vi "LEO_CONTROL.vi"() -> ()   [LabVIEW 2017]
panel:
  in  "SAVE CURRENT IMAGE":bool
  out "Last Action @":string="12:38:13 PM"
  out "Completion Response  2":string=">SmartSEM Remote Control V04.08, 24th July 2009"
  out "Acknowledge Response 2":string="@"
  in  "ANGLE":dbl=45.0 min=0.0 max=360.0
  in  "ON/OFF":bool
  in  "LINE (Y)":i32=384 min=0 max=767
  in  "Y":i32=384 min=0 max=767
  in  "X":i32=512 min=0 max=1023
  in  "MAG":i32=2000 min=5 max=500000
  in  "RATE":i32(ring)=7 items=["1"=1, "2"=2, "3"=3, "4"=4, "5"=5, "6"=6, "7"=7, "8"=8, "9"=9, "10"=10, "11"=11, "12"=12, "13"=13, "14"=14, "15"=15]
  in  "SCAN ROTATION":bool
  in  "CENTER BEAM":bool
  in  "SET NORMAL MODE":bool
  in  "SET LINE MODE":bool
  in  "SET SPOT MODE":bool
  in  "SET MAG":bool
  in  "SET SCAN RATE":bool
  in  "BLANK BEAM":bool
  in  "ABORT":bool
  out "error out 2":errorcluster
  out "Completion Response":string
  out "Acknowledge Response":string
  in  "VER?":bool
  in  "stop":bool
  out "error out":errorcluster={"status"=FALSE, "code"=0, "source"="Response\nindicates valid\n command."}
  in  "VISA resource name":refnum<visa-resource-name>="COM4"
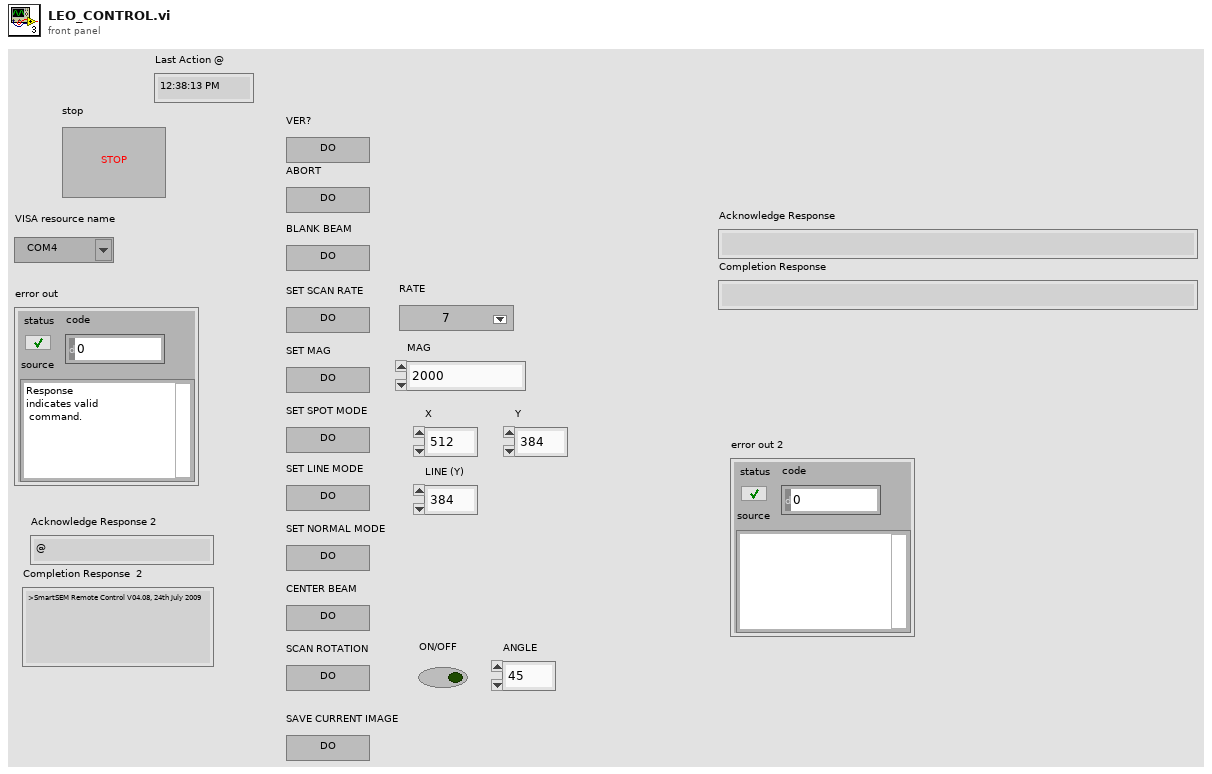
[diagram p1: front panel]
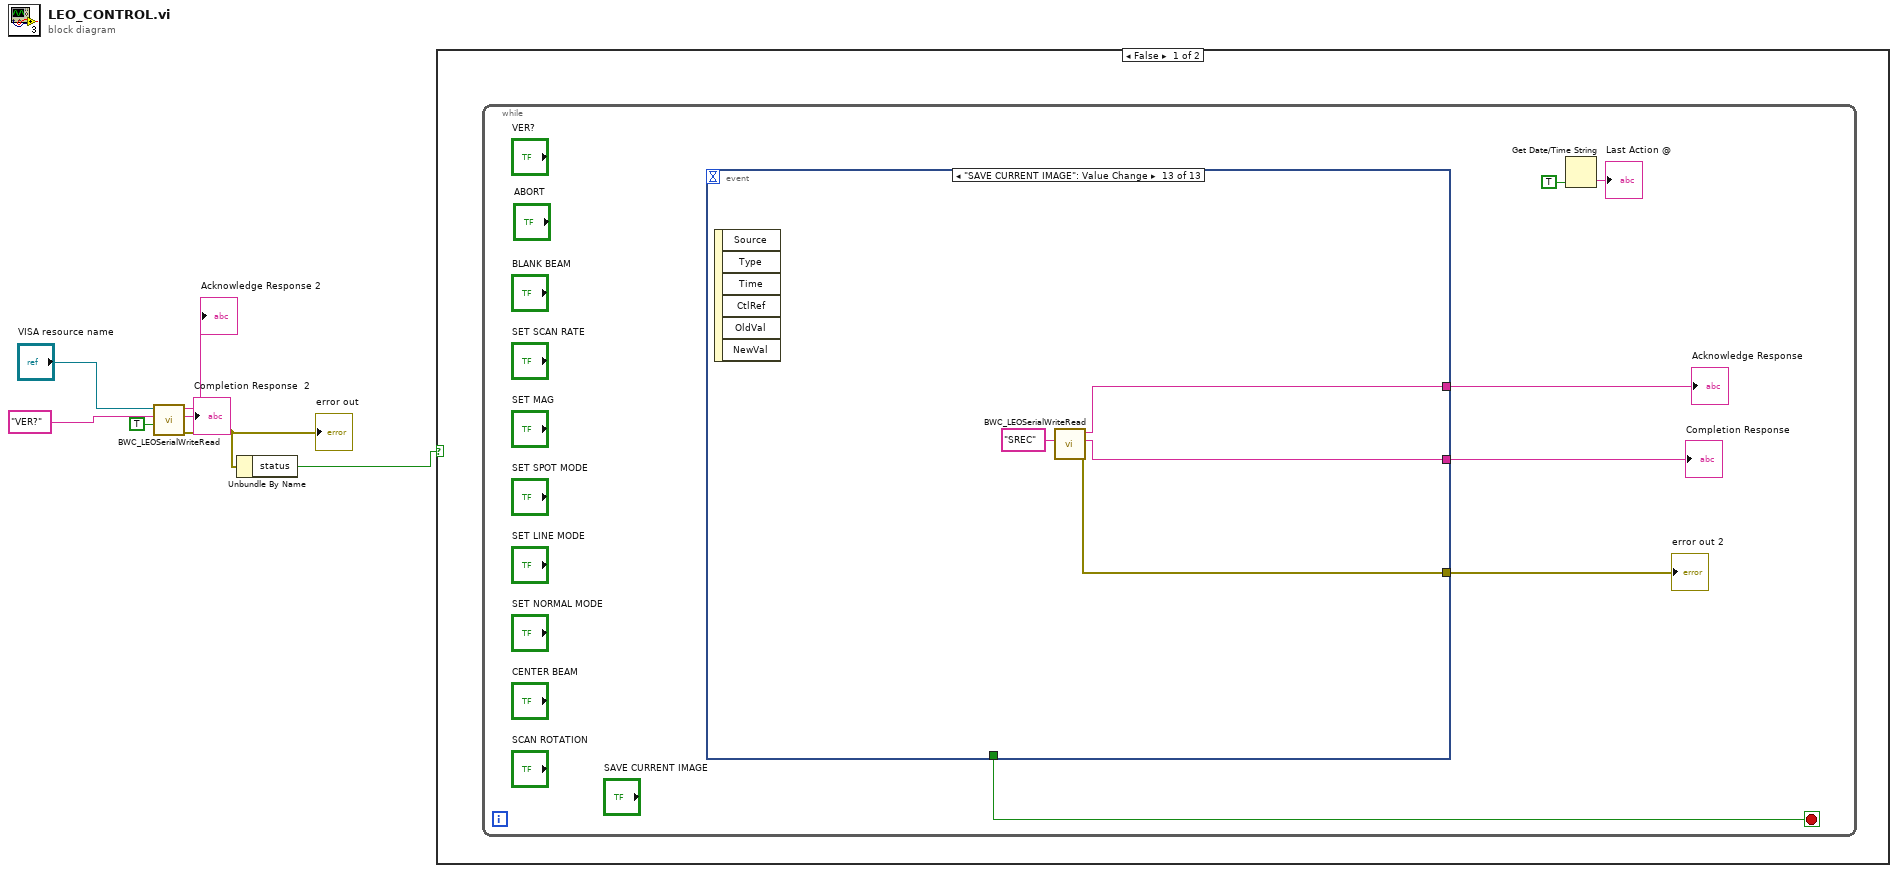
[diagram p0: block diagram]
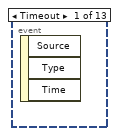
[diagram p2: hidden frame]
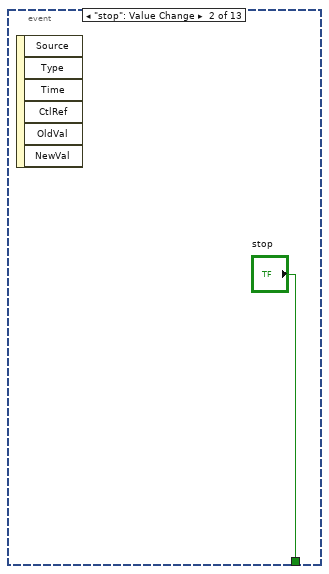
[diagram p3: hidden frame]
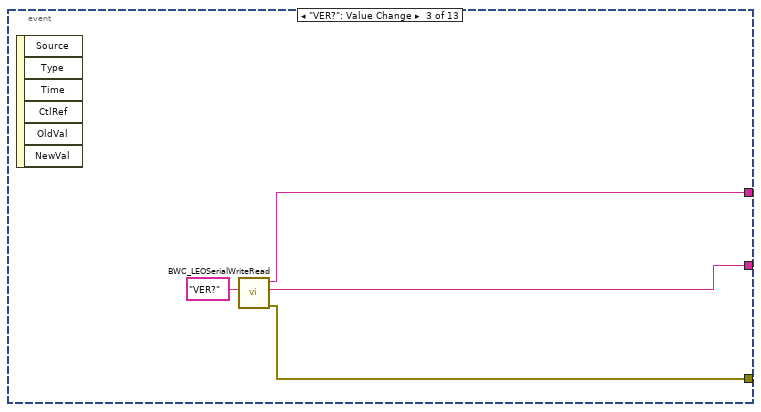
[diagram p4: hidden frame]
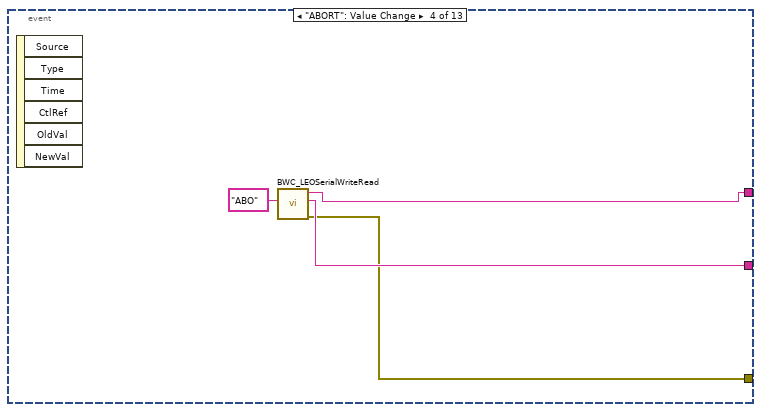
[diagram p5: hidden frame]
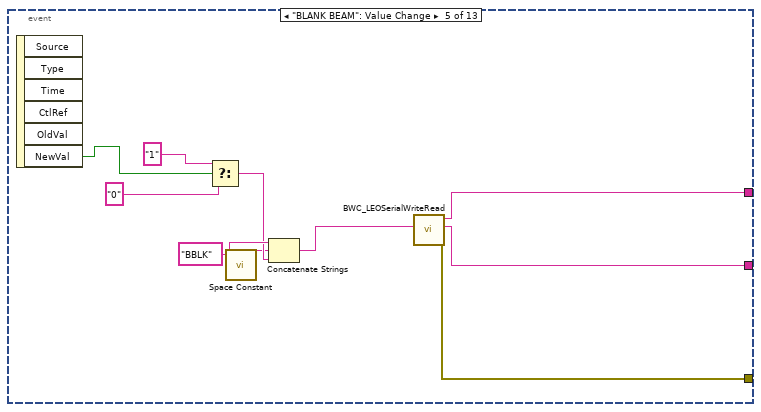
[diagram p6: hidden frame]
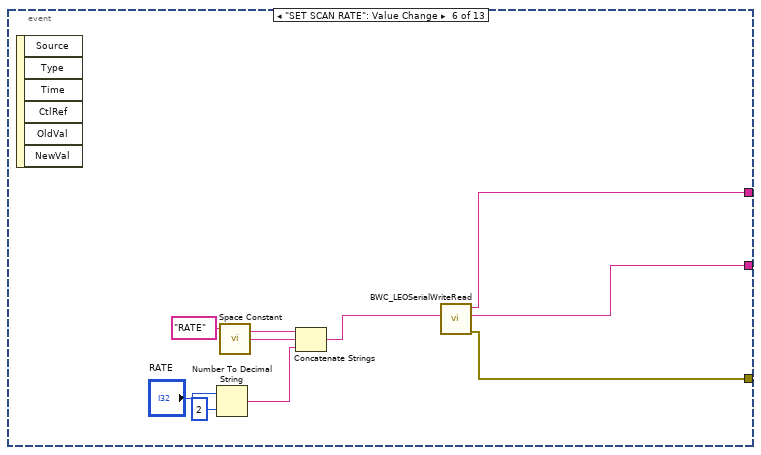
[diagram p7: hidden frame]
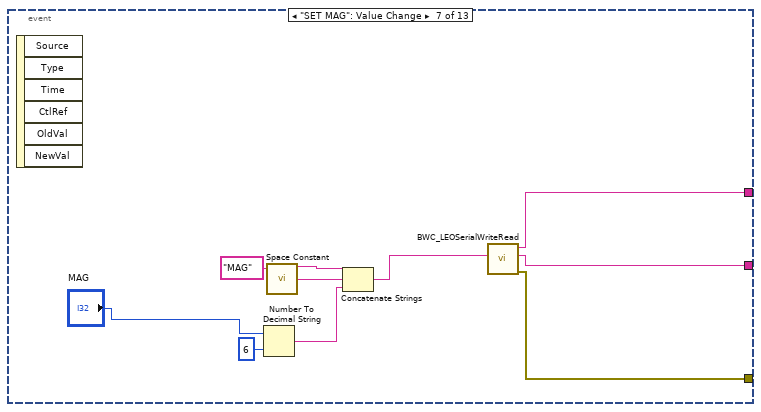
[diagram p8: hidden frame]
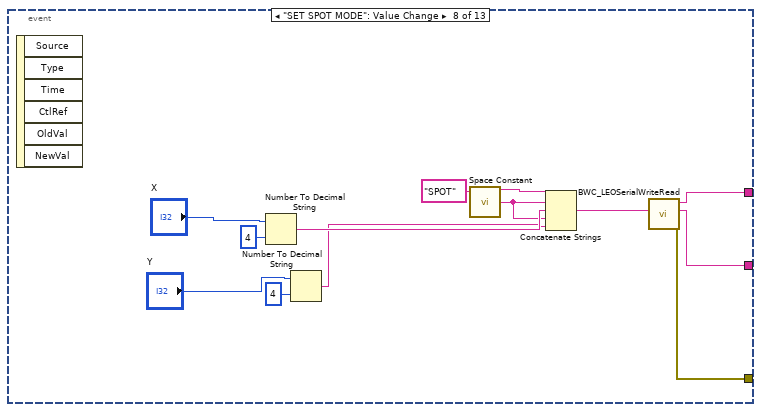
[diagram p9: hidden frame]
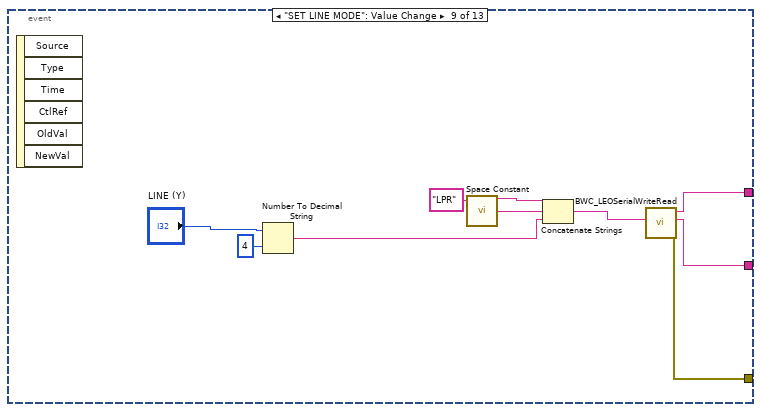
[diagram p10: hidden frame]
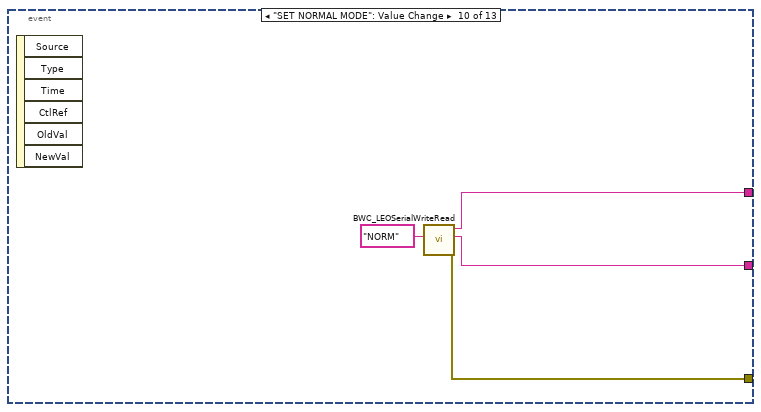
[diagram p11: hidden frame]
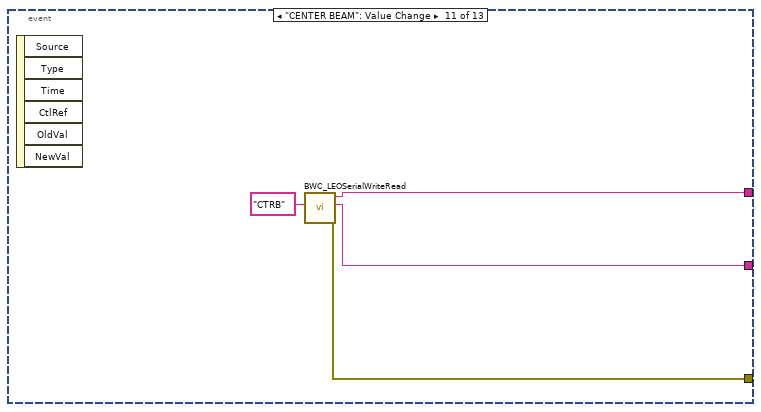
[diagram p12: hidden frame]
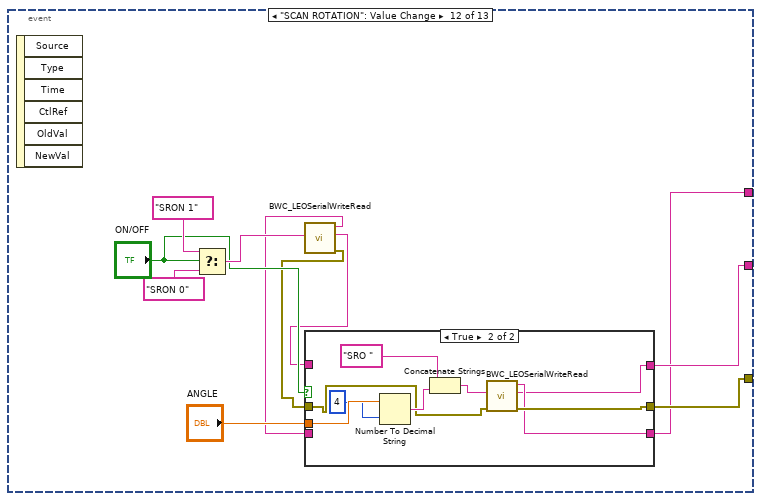
[diagram p13: hidden frame]
diagram:
  n1 = call "BWC_LEOSerialWriteRead.vi"("Perform Two Reads Following Write"=TRUE, "Command To Write"="VER?", "VISA resource name"="VISA resource name") -> ("error out"=w4:errorcluster, "Completion Response"=→"Completion Response  2":string, "Acknowledge Response"=→"Acknowledge Response 2":string)  [unwired: 4 in, 1 out]
  "error out" <- w4
  n2 = Unbundle By Name(w4) -> ("status"=w3:bool)
  n3 = case shown="False" w3 {
    frame False {
      n4 = while {
        stop <- w10 stop-if-true
        n5 = event shown="[12] \"SAVE CURRENT IMAGE\": Value Change" {
          selector: _ -> [_ _ _ _ _ _ _ _ _ _ _ _ _]
          dyn-events: _ -> [_ _ _ _ _ _ _ _ _ _ _ _ _]
          timeout: _ -> [_ _ _ _ _ _ _ _ _ _ _ _ _]
          tunnel: [_ _ w17 w21 w25 w35 w43 w59 w65 w74 w78 w81 w105] -> w13
          tunnel: [_ _ w16 w20 w24 w34 w44 w58 w64 w73 w77 w83 w104] -> w12
          tunnel: [_ _ w15 w19 w23 w33 w42 w57 w63 w72 w76 w84 w103] -> w11
          tunnel: [_ "stop" _ _ _ _ _ _ _ _ _ _ _] -> w10
          event Timeout {
            n6 = event-data() -> ()  [unwired: 1 in, 3 out]
          }
          event "stop": Value Change {
            n7 = event-data() -> ()  [unwired: 1 in, 6 out]
          }
          event "VER?": Value Change {
            n8 = event-data() -> ()  [unwired: 1 in, 6 out]
            n9 = call "BWC_LEOSerialWriteRead.vi"("Command To Write"="VER?") -> ("error out"=w15:errorcluster, "Completion Response"=w16:string, "Acknowledge Response"=w17:string)  [unwired: 6 in, 1 out]
          }
          event "ABORT": Value Change {
            n10 = event-data() -> ()  [unwired: 1 in, 6 out]
            n11 = call "BWC_LEOSerialWriteRead.vi"("Command To Write"="ABO") -> ("error out"=w19:errorcluster, "Completion Response"=w20:string, "Acknowledge Response"=w21:string)  [unwired: 6 in, 1 out]
          }
          event "BLANK BEAM": Value Change {
            n12 = event-data() -> ("NewVal"=w32:bool)  [unwired: 1 in, 5 out]
            n13 = Select(t="1", s=w32, f="0") -> (s? t:f=w28:string)
            n14 = call <vilib>:"Space Constant.vi"() -> ("String"=w27:string)
            n15 = Concatenate Strings("BBLK" ("Command To Write"), w27, w28) -> (w26:string)
            n16 = call "BWC_LEOSerialWriteRead.vi"("Command To Write"=w26) -> ("error out"=w23:errorcluster, "Completion Response"=w24:string, "Acknowledge Response"=w25:string)  [unwired: 6 in, 1 out]
          }
          event "SET SCAN RATE": Value Change {
            n17 = event-data() -> ()  [unwired: 1 in, 6 out]
            n18 = Number To Decimal String(number="RATE", width (-)=i16 2) -> (decimal integer string=w36:string)
            n19 = call <vilib>:"Space Constant.vi"() -> ("String"=w40:string)
            n20 = Concatenate Strings("RATE" ("Command To Write"), w40, w36) -> (w39:string)
            n21 = call "BWC_LEOSerialWriteRead.vi"("Command To Write"=w39) -> ("error out"=w33:errorcluster, "Completion Response"=w34:string, "Acknowledge Response"=w35:string)  [unwired: 6 in, 1 out]
          }
          event "SET MAG": Value Change {
            n22 = event-data() -> ()  [unwired: 1 in, 6 out]
            n23 = Number To Decimal String(number="MAG", width (-)=i16 6) -> (decimal integer string=w50:string)
            n24 = call <vilib>:"Space Constant.vi"() -> ("String"=w48:string)
            n25 = Concatenate Strings("MAG" ("Command To Write"), w48, w50) -> (w49:string)
            n26 = call "BWC_LEOSerialWriteRead.vi"("Command To Write"=w49) -> ("error out"=w42:errorcluster, "Completion Response"=w44:string, "Acknowledge Response"=w43:string)  [unwired: 6 in, 1 out]
          }
          event "SET SPOT MODE": Value Change {
            n27 = event-data() -> ()  [unwired: 1 in, 6 out]
            n28 = Number To Decimal String(number="X", width (-)=i16 4) -> (decimal integer string=w53:string)
            n29 = Number To Decimal String(number="Y", width (-)=i16 4) -> (decimal integer string=w51:string)
            n30 = call <vilib>:"Space Constant.vi"() -> ("String"=w52:string)
            n31 = Concatenate Strings("SPOT" ("Command To Write"), w52, w53, w52, w51) -> (w62:string)
            n32 = call "BWC_LEOSerialWriteRead.vi"("Command To Write"=w62) -> ("error out"=w57:errorcluster, "Completion Response"=w58:string, "Acknowledge Response"=w59:string)  [unwired: 6 in, 1 out]
          }
          event "SET LINE MODE": Value Change {
            n33 = event-data() -> ()  [unwired: 1 in, 6 out]
            n34 = Number To Decimal String(number="LINE (Y)", width (-)=i16 4) -> (decimal integer string=w70:string)
            n35 = call <vilib>:"Space Constant.vi"() -> ("String"=w71:string)
            n36 = Concatenate Strings("LPR" ("Command To Write"), w71, w70) -> (w68:string)
            n37 = call "BWC_LEOSerialWriteRead.vi"("Command To Write"=w68) -> ("error out"=w63:errorcluster, "Completion Response"=w64:string, "Acknowledge Response"=w65:string)  [unwired: 6 in, 1 out]
          }
          event "SET NORMAL MODE": Value Change {
            n38 = event-data() -> ()  [unwired: 1 in, 6 out]
            n39 = call "BWC_LEOSerialWriteRead.vi"("Command To Write"="NORM") -> ("error out"=w72:errorcluster, "Completion Response"=w73:string, "Acknowledge Response"=w74:string)  [unwired: 6 in, 1 out]
          }
          event "CENTER BEAM": Value Change {
            n40 = event-data() -> ()  [unwired: 1 in, 6 out]
            n41 = call "BWC_LEOSerialWriteRead.vi"("Command To Write"="CTRB") -> ("error out"=w76:errorcluster, "Completion Response"=w77:string, "Acknowledge Response"=w78:string)  [unwired: 6 in, 1 out]
          }
          event "SCAN ROTATION": Value Change {
            n42 = event-data() -> ()  [unwired: 1 in, 6 out]
            n43 = Select(t="SRON 1", s="ON/OFF", f="SRON 0") -> (s? t:f=w88:string)
            n44 = call "BWC_LEOSerialWriteRead.vi"("Command To Write"=w88) -> ("error out"=w85:errorcluster, "Completion Response"=w82:string, "Acknowledge Response"=w80:string)  [unwired: 6 in, 1 out]
            n45 = case shown="True" "ON/OFF" {
              tunnel: "ANGLE" -> [_ w102]
              tunnel: w85 -> [w93 w97]
              tunnel: [w93 w96] -> w84
              tunnel: [w92 w94] -> w83
              tunnel: w82 -> [w92 _]
              tunnel: [w91 w95] -> w81
              tunnel: w80 -> [w91 _]
              frame False {
              }
              frame True {
                n46 = Number To Decimal String(number=w102, width (-)=i16 4) -> (decimal integer string=w99:string)
                n47 = Concatenate Strings("SRO " ("string"), w99) -> (w98:string)
                n48 = call "BWC_LEOSerialWriteRead.vi"("error in (no error)"=w97, "Command To Write"=w98) -> ("error out"=w96:errorcluster, "Completion Response"=w94:string, "Acknowledge Response"=w95:string)  [unwired: 5 in, 1 out]
              }
            }
          }
          event "SAVE CURRENT IMAGE": Value Change {
            n49 = event-data() -> ()  [unwired: 1 in, 6 out]
            n50 = call "BWC_LEOSerialWriteRead.vi"("Command To Write"="SREC") -> ("error out"=w103:errorcluster, "Completion Response"=w104:string, "Acknowledge Response"=w105:string)  [unwired: 6 in, 1 out]
          }
        }
        "Acknowledge Response" <- w13
        "Completion Response" <- w12
        "error out 2" <- w11
        n51 = Get Date/Time String(want seconds? (F)=TRUE) -> (time string=→"Last Action @":string)  [unwired: 2 in, 1 out]
      }
    }
    frame True {
    }
  }
